vi "SID_main.vi"() -> ()   [LabVIEW 2018]
doc: "This VI illustrates how to generate and play sine, square, sawtooth and triangle waveforms. You can change the frequency and type of the waveform generated as it plays continuously."
uses:
  SID_voice_reg.ctl
  SID_filter_reg.ctl
  <vilib>/sound2/lvsound2.llb/Sampling Mode.ctl
  <vilib>/sound2/lvsound2.llb/Sound Data Format.ctl
  <vilib>/sound2/lvsound2.llb/Sound Output Set Volume (Single).vi
  <vilib>/sound2/lvsound2.llb/Sound Output Write (DBL Single).vi
panel:
  in  "R":dbl=0.995
  in  "LP":dbl=4000.0
  in  "Volume":dbl=0.5
  in  "delay":dbl=20.0
  out "Filter":T1 {"vol" format="%0.2f"}
  out "VC3":T2 {"ADSR"."S" format="%.2f"}
  out "VC1":T2 {"ADSR"."S" format="%.2f"}
  out "VC2":T2 {"ADSR"."S" format="%.2f"}
  out "VC3":dbl[](graph)
  out "VC2":dbl[](graph)
  out "VC1":dbl[](graph)
  out "Wave":dbl[](graph)
  in  "Stop":bool
  in  "Device ID":u32
  # "Mix"
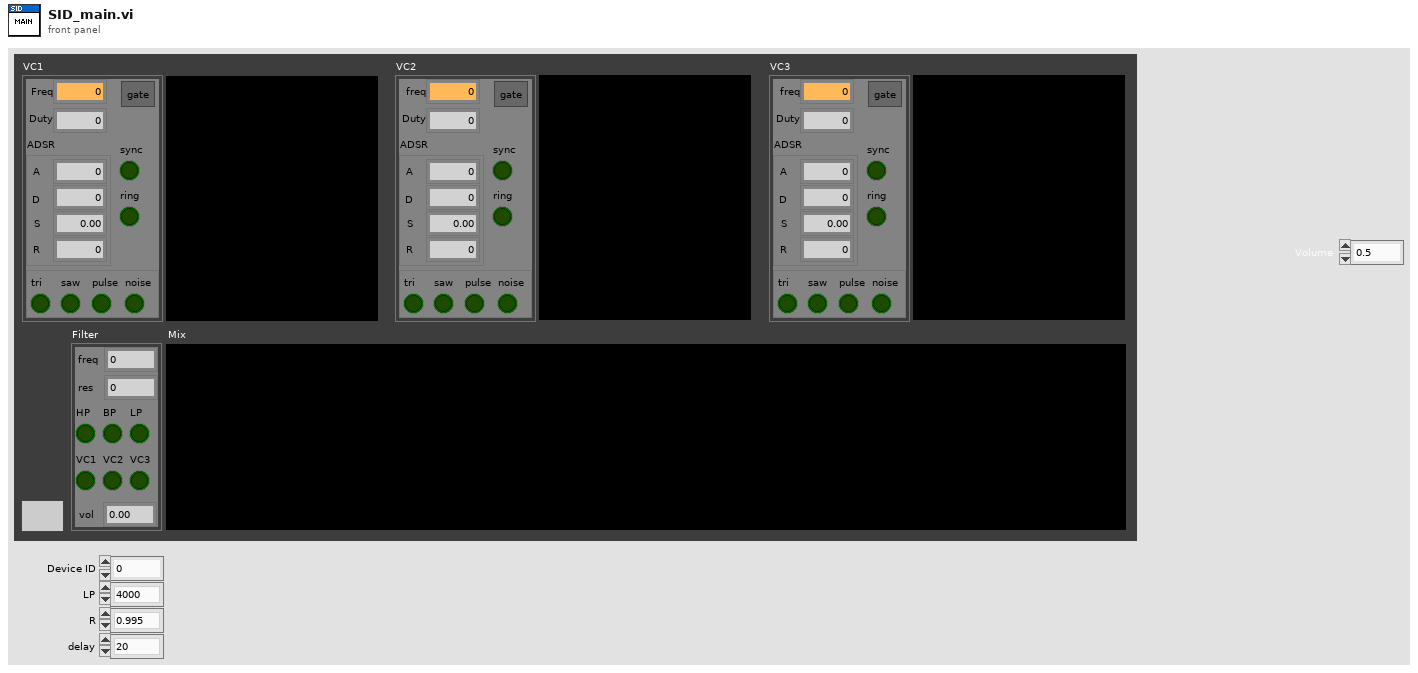
[diagram p1: front panel]
types:
  T1 = typedef "SID_filter_reg.ctl" = cluster{"freq":dbl, "res":dbl, "HP":bool, "BP":bool, "LP":bool, "VC1":bool, "VC2":bool, "VC3":bool, "vol":dbl}
  T2 = typedef "SID_voice_reg.ctl" = cluster{"freq":dbl, "gate":bool, "ADSR":cluster{"A":dbl, "D":dbl, "S":dbl, "R":dbl}, "Duty":dbl, "osc enab":cluster{"tri":bool, "saw":bool, "pulse":bool, "noise":bool}, "sync":bool, "ring":bool}
  T3 = enum16{"idle", "pre-attack", "attack", "pre-decay", "decay", "sustain", "pre-release", "release"}
  T4 = typedef "Sound Data Format.ctl" = cluster{"sample rate (S/s)":dbl, "number of channels":i32, "bits per sample":i32}
  T5 = typedef "Sampling Mode.ctl" = i32
  T6 = typedef "Sound Output Task ID.ctl" = u32
  T7 = cluster{"mod":dbl, "acc":dbl, "counter acc":dbl, "counter":i32}
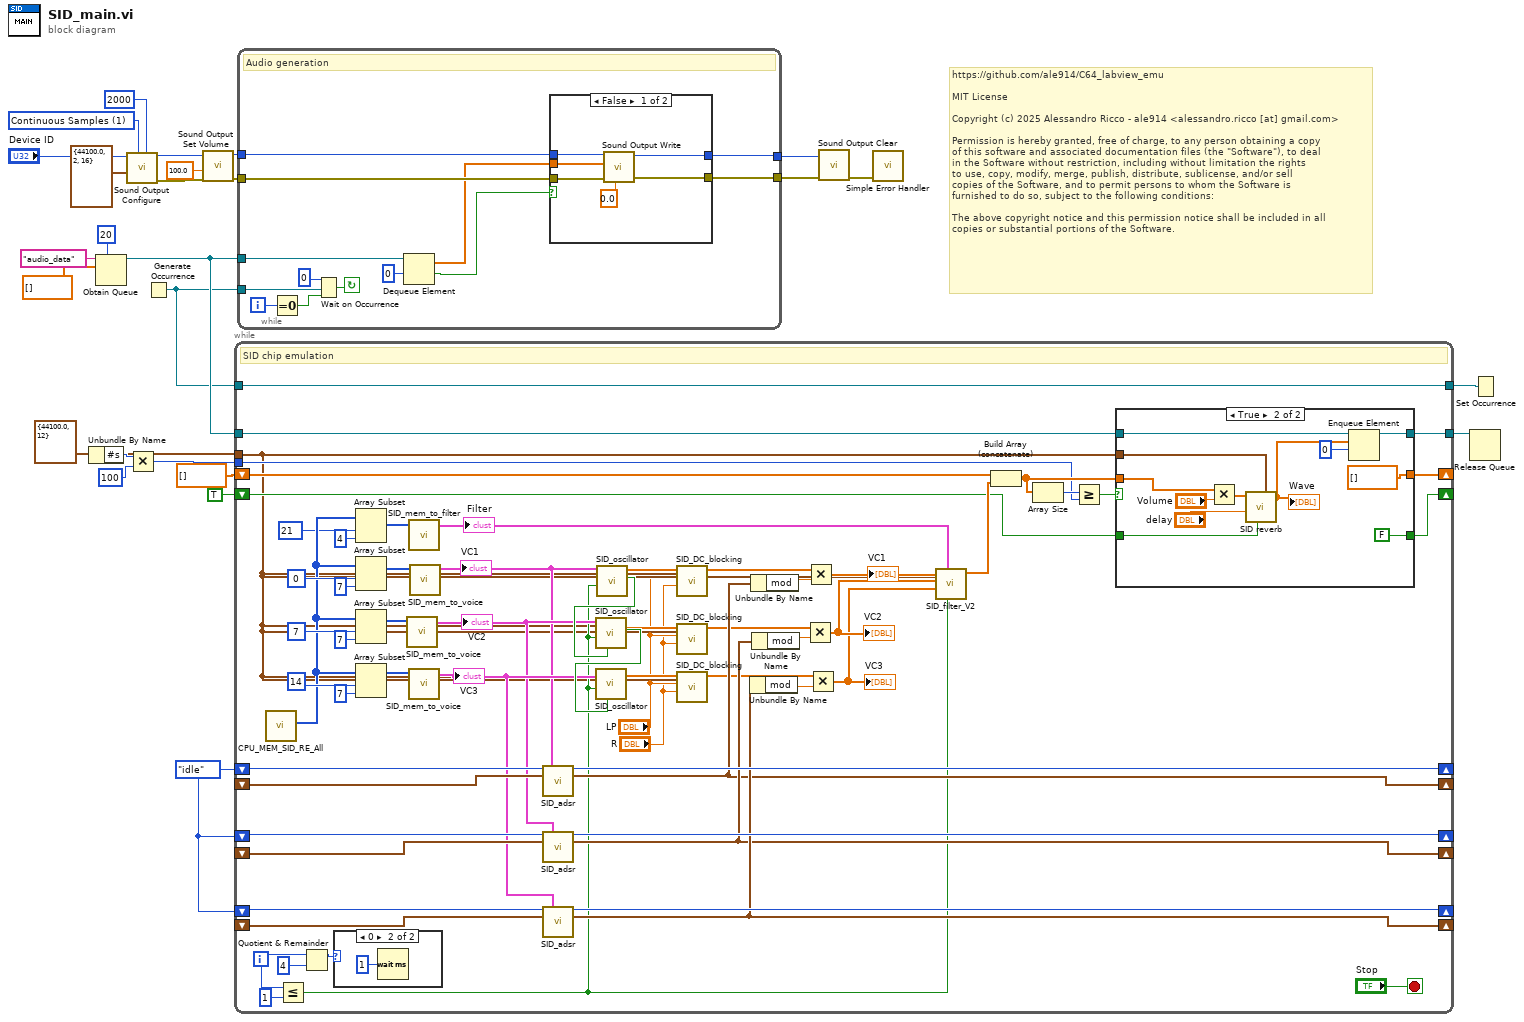
[diagram p0: block diagram]
diagram:
  w6 = cluster{"Fs":dbl, "#s":i32} {"Fs"=44100.0, "#s"=12} ("sampling info")
  w2 = T3."idle"
  w25 = T5 1 items=["Finite Samples", "Continuous Samples"] ("sample mode")
  # "https://github.com/ale914/C64_labview_emu\n\nMIT License\n\nCopyright (c) 2025 Alessandro Ricco - ale914 <alessandro.ricco [at] gmail.com>\n\nPermission is hereby granted, free of charge, to any person obtaining a copy\nof this software and associated documentation files (the \"Software\"), to deal\nin the Software without restriction, including without limitation the rights\nto use, copy, modify, merge, publish, distribute, sublicense, and/or sell\ncopies of the Software, and to permit persons to whom the Software is\nfurnished to do so, subject to the following conditions:\n\nThe above copyright notice and this permission notice shall be included in all\ncopies or substantial portions of the Software."
  n1 = Unbundle By Name(w6) -> ("#s"=w8:i32)
  n2 = Obtain Queue(max queue size (-1, unlimited)=20, name (unnamed)="audio_data", element data type=dbl[] []) -> (queue out=w13:refnum<queue>)  [unwired: 2 in, 2 out]
  n3 = call <vilib>:"Sound Output Configure.vi"("number of samples/ch"=2000 ("Number of Samples/ch"), "sample mode"=w25, "sound format"=T4 {"sample rate (S/s)"=44100.0, "number of channels"=2, "bits per sample"=16} ("Sound Format"), "device ID"="Device ID") -> ("error out"=w22:errorcluster, "task ID"=w20:T6)  [unwired: 6 in]
  n4 = Multiply(x=w8, y=100) -> (x*y=w5:i32)
  n5 = Generate Occurrence() -> (w4:refnum<k4>)
  n6 = call-poly <vilib>:"Sound Output Set Volume.vi"("error in (no error)"=w22, "volume"=100.0, "task ID"=w20) -> ("error out"=w18:errorcluster, "task ID out"=w19:T6)  [unwired: 7 in]
  n7 = while {
    shift-right: [w62] -> _
    shift-left: _ -> [w80]
    shift-right: [w79] -> _
    shift-left: w2 -> [w81]
    tunnel: w4 -> [w90]
    tunnel: [w90] -> w15
    tunnel: w13 -> [w88]
    tunnel: [w87] -> w12
    shift-right: [w82] -> _
    shift-left: dbl[] [] -> [w86]
    shift-right: [w63] -> _
    shift-left: _ -> [w77]
    shift-right: [w76] -> _
    shift-left: w2 -> [w78]
    tunnel: w6 -> [w31]
    shift-right: [w64] -> _
    shift-left: _ -> [w74]
    shift-right: [w75] -> _
    shift-left: w2 -> [w73]
    tunnel: w5 -> [w72]
    shift-right: [w36] -> _
    shift-left: TRUE -> [w37]
    i -> [w60]
    stop <- "Stop" stop-if-true
    # "SID chip emulation"
    n8 = call "CPU_MEM_SID_RE_All.vi"() -> ("mem"=w45:u8[])  [unwired: 11 in]
    n9 = Less Or Equal?(x=w60, y=1) -> (x <= y?=w39:bool)
    n10 = Quotient & Remainder(x=w60, y=4) -> (x-y*floor(x/y)=w58:i32)  [unwired: 1 out]
    n11 = case shown="0" w58 {
      frame Default {
      }
      frame 0 {
        n12 = Wait (ms)(milliseconds to wait=u32 1) -> ()  [unwired: 1 out]
      }
    }
    n13 = Array Subset(array=w45, index=21 ("address"), length=4) -> (w43:u8[])
    n14 = Array Subset(array=w45, index=0 ("address"), length=7) -> (w54:u8[])
    n15 = Array Subset(array=w45, index=7 ("address"), length=7) -> (w48:u8[])
    n16 = Array Subset(array=w45, index=14 ("address"), length=7) -> (w47:u8[])
    n17 = call "SID_mem_to_voice.vi"("mem"=w48) -> ("VC"=w66:T2)  [unwired: 10 in]
    "VC2" <- w66
    n18 = call "SID_mem_to_filter.vi"("mem"=w43) -> ("filter reg"=w56:T1)  [unwired: 10 in]
    "Filter" <- w56
    n19 = call "SID_mem_to_voice.vi"("mem"=w47) -> ("VC"=w67:T2)  [unwired: 10 in]
    "VC3" <- w67
    n20 = call "SID_mem_to_voice.vi"("mem"=w54) -> ("VC"=w57:T2)  [unwired: 10 in]
    "VC1" <- w57
    n21 = call "SID_adsr.vi"("status in"=w81, "Reg"=w57, "acc in"=w80) -> ("status out"=w79:T3, "acc out"=w62:T7)  [unwired: 11 in]
    n22 = call "SID_adsr.vi"("status in"=w78, "Reg"=w66, "acc in"=w77) -> ("status out"=w76:T3, "acc out"=w63:T7)  [unwired: 11 in]
    n23 = call "SID_adsr.vi"("status in"=w73, "Reg"=w67, "acc in"=w74) -> ("status out"=w75:T3, "acc out"=w64:T7)  [unwired: 11 in]
    n24 = call "SID_oscillator.vi"("sampling info"=w31, "Reg"=w57, "reset phase"=w39) -> ("MSB out"=w69:bool, "wave"=w28:dbl[])  [unwired: 7 in]
    n25 = call "SID_oscillator.vi"("sampling info"=w31, "MSB in"=w69, "Reg"=w66, "reset phase"=w39) -> ("MSB out"=w68:bool, "wave"=w35:dbl[])  [unwired: 6 in]
    n26 = call "SID_oscillator.vi"("sampling info"=w31, "MSB in"=w68, "Reg"=w67, "reset phase"=w39) -> ("wave"=w33:dbl[])  [unwired: 6 in, 1 out]
    n27 = call "SID_DC_blocking.vi"("sampling info"=w31, "R"="R", "low pass"="LP", "wave in"=w28) -> ("wave out"=w27:dbl[])  [unwired: 7 in]
    n28 = call "SID_DC_blocking.vi"("sampling info"=w31, "R"="R", "low pass"="LP", "wave in"=w35) -> ("wave out"=w34:dbl[])  [unwired: 7 in]
    n29 = call "SID_DC_blocking.vi"("sampling info"=w31, "R"="R", "low pass"="LP", "wave in"=w33) -> ("wave out"=w32:dbl[])  [unwired: 7 in]
    n30 = Unbundle By Name(w64) -> ("mod"=w40:dbl)
    n31 = Unbundle By Name(w62) -> ("mod"=w41:dbl)
    n32 = Unbundle By Name(w63) -> ("mod"=w42:dbl)
    n33 = Multiply(x=w34, y=w42) -> (x*y=w71:dbl[])
    "VC2" <- w71
    n34 = Multiply(x=w27, y=w41) -> (x*y=w61:dbl[])
    "VC1" <- w61
    n35 = Multiply(x=w32, y=w40) -> (x*y=w65:dbl[])
    "VC3" <- w65
    n36 = call "SID_filter_V2.vi"("sampling info"=w31, "reset"=w39, "filter"=w56, "VC3"=w65, "VC2"=w71, "VC1"=w61) -> ("out"=w38:dbl[])  [unwired: 5 in]
    n37 = Build Array (concatenate)(w86, w38) -> (w83:dbl[])
    n38 = Array Size(array=w83) -> (size(s)=w85:i32)
    n39 = Greater Or Equal?(x=w85, y=w72) -> (x >= y?=w84:bool)
    n40 = case shown="True" w84 {
      tunnel: w88 -> [w93 w106]
      tunnel: [w93 w105] -> w87
      tunnel: w83 -> [w94 w101]
      tunnel: [w94 dbl[] []] -> w82
      tunnel: w31 -> [_ w97]
      tunnel: w37 -> [w92 w96]
      tunnel: [w92 FALSE] -> w36
      frame False {
      }
      frame True {
        n41 = Multiply(x=w101, y="Volume") -> (x*y=w100:dbl[])
        n42 = call "SID reverb.vi"("sampling info"=w97, "reset"=w96, "delay"="delay", "wave in"=w100) -> ("wave out"=w99:dbl[])  [unwired: 7 in]
        "Wave" <- w99
        n43 = Enqueue Element(queue=w106, element=w99, timeout in ms (-1)=0) -> (queue out=w105:refnum<queue>)  [unwired: 1 in, 2 out]
      }
    }
  }
  n44 = while {
    tunnel: w19 -> [w114]
    tunnel: w18 -> [w115]
    tunnel: [w111] -> w17
    tunnel: [w110] -> w16
    tunnel: w4 -> [w119]
    tunnel: w13 -> [w112]
    i -> [w116]
    stop <- w117 continue-if-true
    # "Audio generation"
    n45 = Equal To 0?(x=w116) -> (x = 0?=w109:bool)
    n46 = Wait on Occurrence(1:w109, 2:w119, 3:0 ("ms timeout (-1)")) -> (0:w117:bool)
    n47 = Dequeue Element(queue=w112, timeout in ms (-1)=0) -> (element=w108:dbl[], timed out?=w107:bool)  [unwired: 1 in, 2 out]
    n48 = case shown="False" w107 {
      tunnel: w115 -> [w125 w126]
      tunnel: w114 -> [w124 w127]
      tunnel: [w122 w127] -> w111
      tunnel: [w121 w126] -> w110
      tunnel: w108 -> [w120 _]
      frame False {
        n49 = call-poly <vilib>:"Sound Output Write.vi"("timeout (sec)"=0.0, "error in (no error)"=w125, "data"=w120, "task ID"=w124) -> ("error out"=w121:errorcluster, "task ID out"=w122:T6)  [unwired: 6 in]
      }
      frame True {
      }
    }
  }
  n50 = call <vilib>:"Sound Output Clear.vi"("error in (no error)"=w16, "task ID"=w17) -> ("error out"=w23:errorcluster)  [unwired: 9 in]
  n51 = call <vilib>:"Simple Error Handler.vi"("error in (no error)"=w23) -> ()  [unwired: 4 in, 5 out]
  n52 = Release Queue(queue=w12) -> ()  [unwired: 2 in, 3 out]
  n53 = Set Occurrence(w15) -> ()
